vi "GetGcolor.vi"(0 "sdf in":string) -> (1 "color":cluster{dbl, dbl, dbl, dbl}, 2 "sdf out":string)   [LabVIEW 2012]
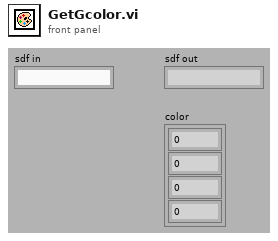
[diagram p1: front panel]
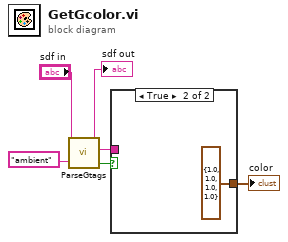
[diagram p0: block diagram]
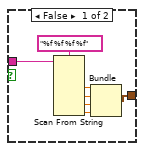
[diagram p2: hidden frame]
diagram:
  n1 = call <userlib>:"ParseGtags.vi"("tag"="ambient", "urdf in"="sdf in") -> ("not found"=w1:bool, "contents"=w4:string, "urdf out"=→"sdf out":string)  [unwired: 1 out]
  n2 = case shown="True" w1 {
    tunnel: [w13 cluster{dbl, dbl, dbl, dbl} {1.0, 1.0, 1.0, 1.0}] -> w6
    tunnel: w4 -> [w12 _]
    frame False {
      n3 = Scan From String(format string="%f %f %f %f", input string=w12) -> (output 1=w8:dbl, output 2=w11:dbl, output 3=w10:dbl, output 4=w9:dbl)  [unwired: 6 in, 3 out]
      n4 = Bundle(w8, w11, w10, w9) -> (w13:cluster{dbl, dbl, dbl, dbl})  [unwired: 1 in]
    }
    frame True {
    }
  }
  "color" <- w6
